vi "com port send response test array.vi"(7 "CMD array":T1[](array[typedef]), 8 "error in (no error)":errorcluster, 9 "Log in":string, 10 "PassFail_In":bool=TRUE, 11 "VISA Send port in":refnum<visa-resource-name>) -> (0 "error out":errorcluster, 1 "Log out":string, 2 "PassFail_Out":bool, 3 "VISA Send port out":refnum<visa-resource-name>)   [LabVIEW 2013]
uses:
  AT cmd list.ctl
  Test Support VI/String compare type.ctl
panel:
  out "Response":string
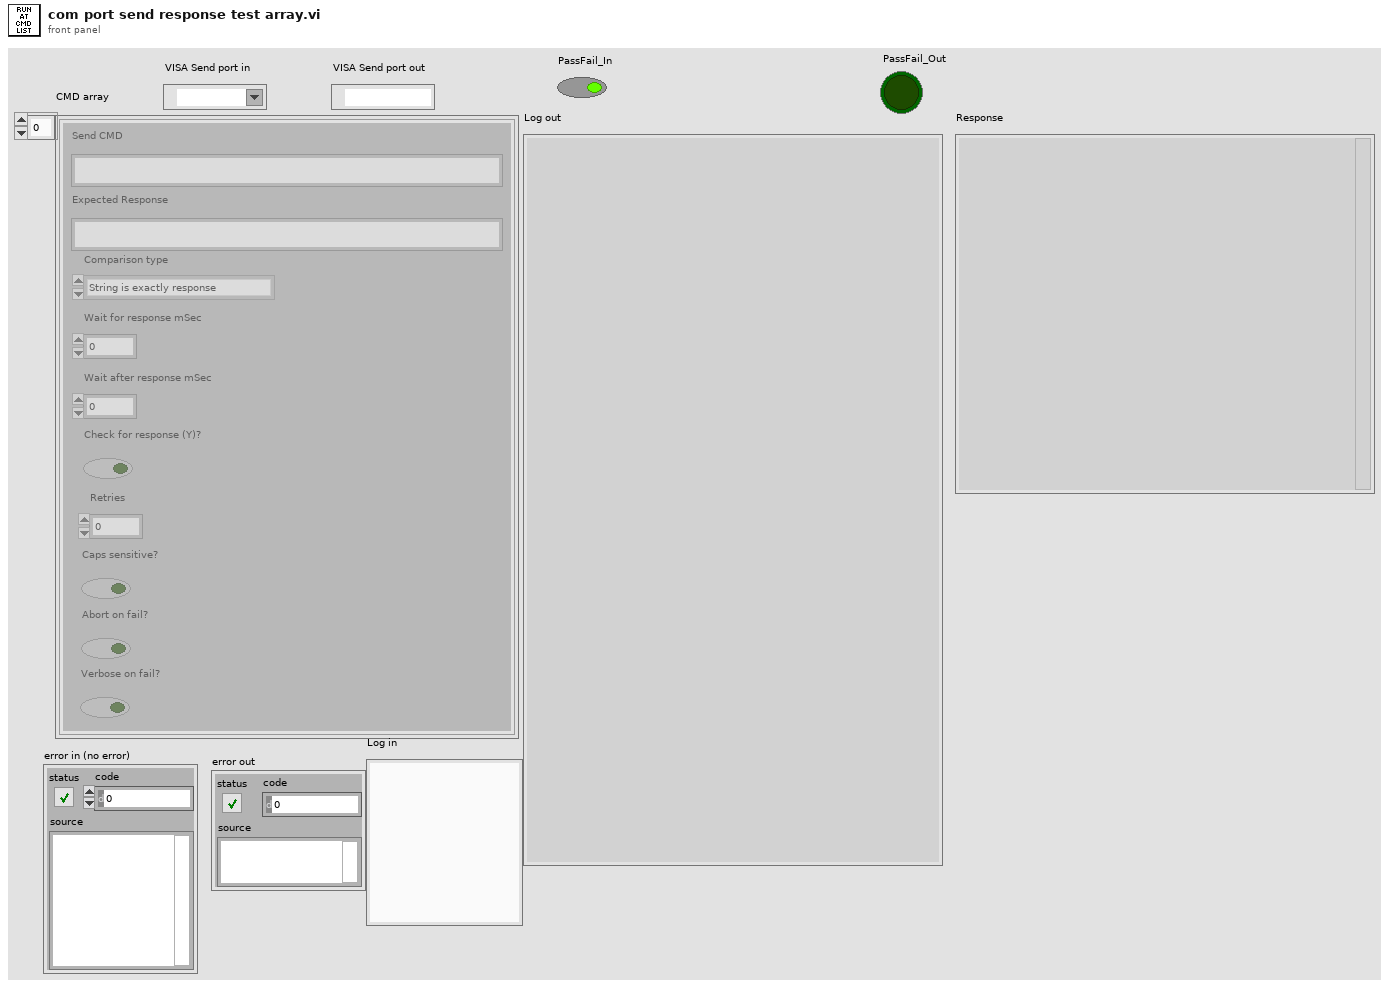
[diagram p1: front panel]
types:
  T1 = typedef "AT cmd list.ctl" = cluster{"Send CMD":string, "Expected Response":string, "Comparison type":T2, "Wait for response mSec":dbl, "Wait after response mSec":dbl, "Check for response (Y)?":bool, "Retries":dbl, "Caps sensitive?":bool, "Abort on fail?":bool, "Verbose on fail?":bool}
  T2 = typedef "String compare type.ctl" = enum16{"String is exactly response", "String in response somewhere", "String not in response"}
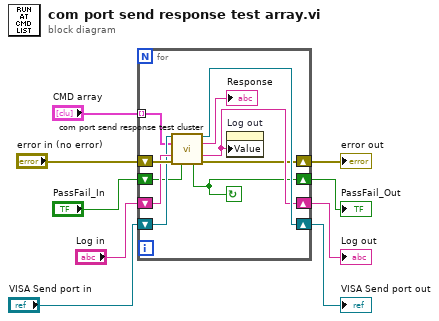
[diagram p0: block diagram]
diagram:
  n1 = for {
    tunnel: "CMD array" -> [w12] mode=indexing
    shift-right: [w11] -> w7
    shift-left: "error in (no error)" -> [w19]
    shift-right: [w14] -> w6
    shift-left: "Log in" -> [w18]
    shift-right: [w17] -> w1
    shift-left: "VISA Send port in" -> [w16]
    shift-right: [w10] -> w4
    shift-left: "PassFail_In" -> [w13]
    stop <- w10 continue-if-true
    n2 = call "com port send response test cluster.vi"("VISA Send port"=w16, "AT CMD List"=w12, "Log in"=w18, "error in (no error)"=w19, "PassFail_In"=w13) -> ("VISA Send port out"=w17:refnum<visa-resource-name>, "Response"=→"Response":string, "Log out"=w14:string, "PassFail_Out"=w10:bool, "error out"=w11:errorcluster)  [unwired: 6 in]
    n3 = property on="Log out" class="Str"("Value"=w14) -> ()  [unwired: 2 in, 2 out]
  }
  "error out" <- w7
  "Log out" <- w6
  "PassFail_Out" <- w4
  "VISA Send port out" <- w1
